vi "newmark_move.vi"(6 "Axis enable":bool[](array[boolean]), 8 "error in":errorcluster, 9 "Axis positions":dbl[](array[numeric])=[0.0, 0.0], 10 "Absolute":bool=TRUE, 11 "VISA Refnum in":refnum<visa-resource-name>) -> (0 "error out":errorcluster, 1 "read string":string, 3 "VISA Refnum out":refnum<visa-resource-name>)   [LabVIEW 2012]
panel:
  # "(degrees)"
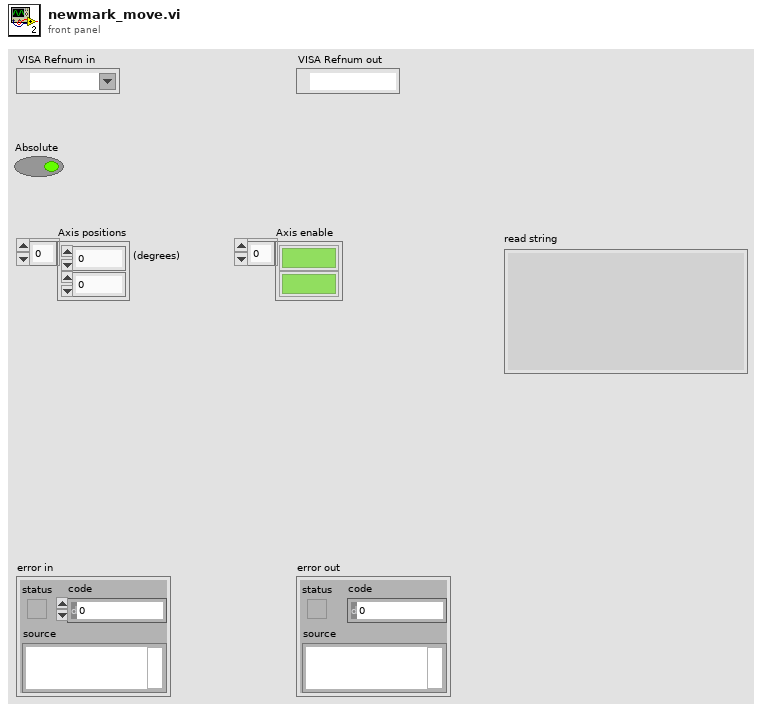
[diagram p1: front panel]
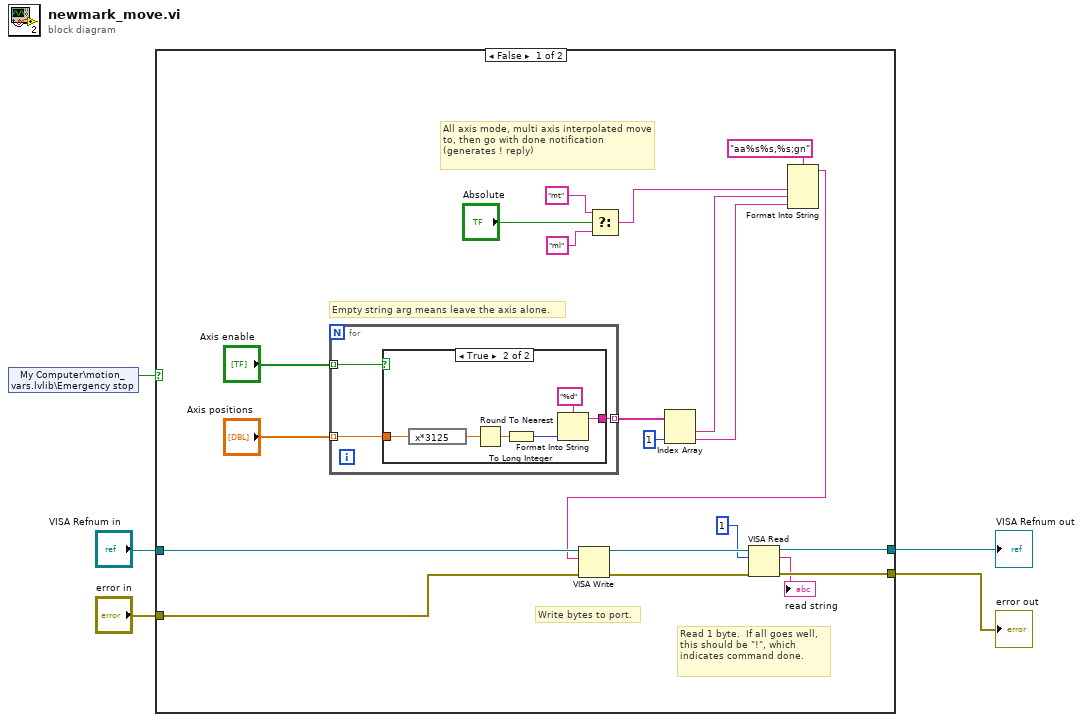
[diagram p0: block diagram]
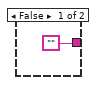
[diagram p2: hidden frame]
diagram:
  n1 = shared-variable "My Computer\\motion_vars.lvlib\\Emergency stop"() -> (w1:bool)  [unwired: 1 in, 1 out]
  n2 = case shown="False" w1 {
    tunnel: [w25 w37] -> w5
    tunnel: [w24 w36] -> w4
    tunnel: "VISA Refnum in" -> [w23 w37]
    tunnel: "error in" -> [w22 w36]
    frame False {
      # "Empty string arg means leave the axis alone."
      # "Read 1 byte.  If all goes well, this should be \"!\", which indicates command done."
      # "All axis mode, multi axis interpolated move to, then go with done notification (generates ! reply)"
      # "Write bytes to port."
      n3 = for {
        tunnel: "Axis positions" -> [w28] mode=indexing
        tunnel: [w27] -> w12 mode=indexing
        tunnel: "Axis enable" -> [w26] mode=indexing
        n4 = case shown="True" w26 {
          tunnel: w28 -> [_ w34]
          tunnel: ["" w31] -> w27
          frame False {
          }
          frame True {
            n5 = expression code="x*3125"(w34) -> (w33:dbl)
            n6 = Round To Nearest(number=w33) -> (nearest integer value=w32:dbl)
            n7 = To Long Integer(number=w32) -> (32bit integer=w30:i32)
            n8 = Format Into String(format string="%d", w30) -> (resulting string=w31:string)  [unwired: 2 in, 1 out]
          }
        }
      }
      n9 = Select(t="mt" ("string"), s="Absolute", f="ml" ("string")) -> (s? t:f=w9:string)
      n10 = Index Array(array=w12, index #2=1 ("index")) -> (element #1=w8:string, element #2=w7:string)  [unwired: 1 in]
      n11 = Format Into String(format string="aa%s%s,%s;gn", w9, w8, w7) -> (resulting string=w10:string)  [unwired: 2 in, 1 out]
      n12 = VISA Write(VISA resource name=w23, write buffer=w10, error in (no error)=w22) -> (VISA resource name out=w18:refnum<visa-resource-name>, error out=w17:errorcluster)  [unwired: 1 out]
      n13 = VISA Read(VISA resource name=w18, byte count=u32 1, error in (no error)=w17) -> (VISA resource name out=w25:refnum<visa-resource-name>, read buffer=→"read string":string, error out=w24:errorcluster)  [unwired: 1 out]
    }
    frame True {
    }
  }
  "VISA Refnum out" <- w5
  "error out" <- w4
